vi "Read Rank.vi"(8 "error in (no error)":errorcluster, 11 "Tag in":refnum<class "Tag.lvclass">) -> (0 "error out":errorcluster, 2 "Rank":u8, 3 "Tag out":refnum<class "Tag.lvclass">)   [LabVIEW 2018, in "Tag Engine.lvlib" / "Tag.lvclass"]
doc: "_SubVI_"
uses:
  Tag.lvclass
  Tag.lvclass/Tag.ctl
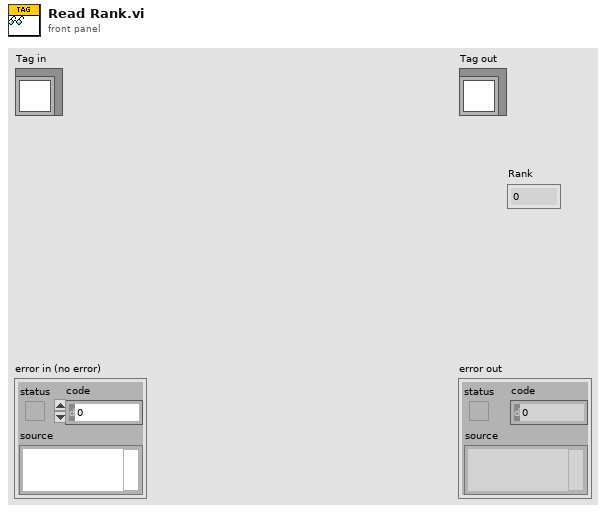
[diagram p1: front panel]
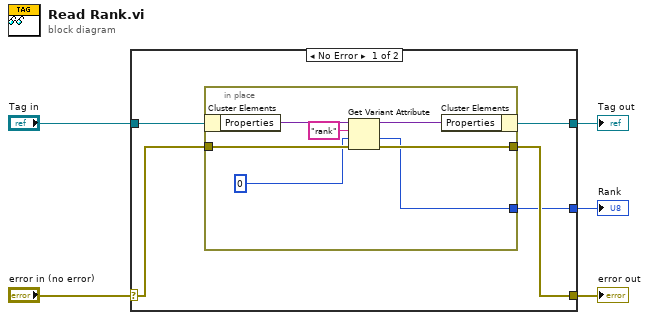
[diagram p0: block diagram]
diagram:
  n1 = case shown="No Error" "error in (no error)" {
    selector: "error in (no error)" -> [w8 w18]
    tunnel: [w7 w18] -> w4
    tunnel: [w9 w19] -> w2
    tunnel: "Tag in" -> [w10 w19]
    tunnel: [w6 _] -> w1
    frame No Error {
      n2 = in-place {
        in-place-border: w8 -> [w14]
        in-place-border: [w13] -> w7
        in-place-border: [w12] -> w6
        n3 = in-place-cluster #1(w10) -> ("Properties"=w17:variant)
        n4 = Get Variant Attribute(Variant=w17, name="rank", default value (empty Variant)=u8 0, error in=w14) -> (duplicate Variant=w15:variant, value=w12:u8, error out=w13:errorcluster)  [unwired: 1 out]
        n5 = in-place-cluster #1("Properties"=w15) -> (w9:refnum<class "Tag.lvclass">)
      }
    }
    frame Error {
    }
  }
  "error out" <- w4
  "Tag out" <- w2
  "Rank" <- w1
